vi "Configure Preset Action (AO).vi"(0 "VISA resource name":refnum<visa-resource-name>, 1 "Channel (0001)":string="0001", 2 "Value at power on (1:Preset Value)":i32(ring)=1 items=["Last Value", "Preset Value"], 3 "Value on error (1:Preset Value)":i32(ring)=1 items=["Last Value", "Preset Value"], 4 "Value at stopping record (1:Preset Value)":i32(ring)=1 items=["Last Value", "Preset Value"], 5 "error in (no error)":errorcluster) -> (14 "VISA resource name out":refnum<visa-resource-name>, 19 "error out":errorcluster)   [LabVIEW 2020, in "Yokogawa GX Series.lvlib"]
doc: "Sets preset action of AO channel.\n\nCommand: SPresetAO"
uses:
  <instrlib>/Yokogawa GX Series/Yokogawa GX Series.lvlib
panel:
  out "Channel":string
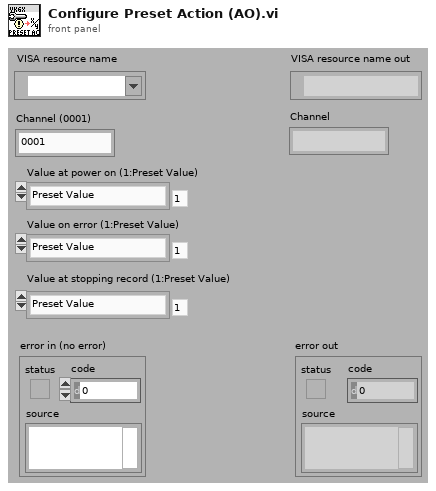
[diagram p1: front panel]
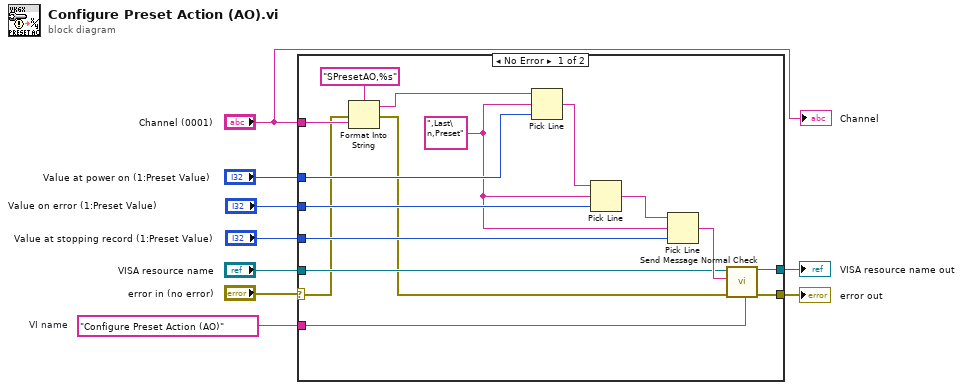
[diagram p0: block diagram]
diagram:
  w8 = "Configure Preset Action (AO)"  # VI name
  n1 = case shown="No Error" "error in (no error)" {
    selector: "error in (no error)" -> [w13 w26]
    tunnel: "VISA resource name" -> [w16 w27]
    tunnel: w8 -> [w15 _]
    tunnel: [w25 w27] -> w3
    tunnel: [w24 w26] -> w2
    tunnel: "Value at stopping record (1:Preset Value)" -> [w21 _]
    tunnel: "Value at power on (1:Preset Value)" -> [w23 _]
    tunnel: "Value on error (1:Preset Value)" -> [w22 _]
    tunnel: "Channel (0001)" -> [w14 _]
    frame No Error {
      w18 = ",Last\n,Preset"
      n2 = Format Into String(format string="SPresetAO,%s", error in=w13, w14) -> (resulting string=w10:string, error out=w12:errorcluster)  [unwired: 1 in]
      n3 = Pick Line(string ("")=w10, multi-line string=w18, line index=w23) -> (output string=w20:string)
      n4 = Pick Line(string ("")=w20, multi-line string=w18, line index=w22) -> (output string=w19:string)
      n5 = Pick Line(string ("")=w19, multi-line string=w18, line index=w21) -> (output string=w17:string)
      n6 = call <instrlib>:"Send Message Normal Check.vi"("Source (\"\")"=w15, "error in (no error)"=w12, "Send Message (\"\")"=w17, "VISA resource name"=w16) -> ("error out"=w24:errorcluster, "VISA resource name out"=w25:refnum<visa-resource-name>)  [unwired: 2 in, 4 out]
    }
    frame Error {
    }
  }
  "error out" <- w2
  "VISA resource name out" <- w3
  "Channel" <- "Channel (0001)"
